vi "SubSystems.vi"(8 "error in":errorcluster) -> ()   [LabVIEW 2025]
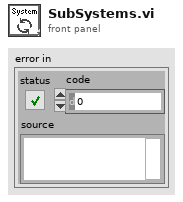
[diagram p1: front panel]
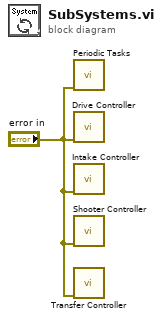
[diagram p0: block diagram]
diagram:
  n1 = call "Periodic Tasks.vi"("error in"="error in") -> ()  [unwired: 1 in, 10 out]
  n2 = call "Drive Controller.vi"("error in"="error in") -> ()  [unwired: 11 in]
  n3 = call "Intake Controller.vi"("error in"="error in") -> ()  [unwired: 11 in]
  n4 = call "Shooter Controller.vi"("error in"="error in") -> ()  [unwired: 11 in]
  n5 = call "Transfer Controller.vi"("error in"="error in") -> ()  [unwired: 11 in]
